vi "Scan action.vi"(0 "Index":i32, 1 "Channels: AO":T1={"AO amp (V)"=[0.002, 0.002, 0.002, 0.002, 0.002, 0.002, 0.002, 0.002], "AO DC (V)"=[0.0, 0.0, 0.0, 0.0, 0.0, 0.0, 0.0, 0.0], "AO f (Hz)"=[15.1, 15.11, 15.12, 15.13, 15.14, 15.15, 15.16, 15.17], "AO phi (deg)"=[0.0, 10.0, 20.0, 30.0, 40.0, 50.0, 60.0, 70.0], "function"=[enum."Sine Wave", enum."Sine Wave", enum."Sine Wave", enum."Sine Wave", enum."Sine Wave", enum."Sine Wave", enum."Sine Wave", enum."Sine Wave"]} {"AO f (Hz)" min=0.001 max=10000.0; "AO DC (V)" format="%#_6p"; "AO amp (V)" format="%#_6p"}, 2 "Scan control":T9=enum."DSA_Vamp", 3 "Scan Parameters":T8={"DAQ Channel"=2, "Label"="\nscaledVsg1=", "Start"=0.14, "End"=-0.060000000000000005, "Step"=-0.060000000000000005, "Rate"=-0.060000000000000005, "VISA resource name"=""} {"Rate" format="%.2f"; "Step" format="%#_6p"; "End" format="%#_6p"; "Start" format="%#_6p"}, 4 "Comments":string) -> (5 "Comments out":string, 6 "Channels: AO":T1={"AO amp (V)"=[0.002, 0.002, 0.002, 0.002, 0.002, 0.002, 0.002, 0.002], "AO DC (V)"=[0.0, 0.0, 0.0, 0.0, 0.0, 0.0, 0.0, 0.0], "AO f (Hz)"=[15.1, 15.11, 15.12, 15.13, 15.14, 15.15, 15.16, 15.17], "AO phi (deg)"=[0.0, 10.0, 20.0, 30.0, 40.0, 50.0, 60.0, 70.0], "function"=[enum."Sine Wave", enum."Sine Wave", enum."Sine Wave", enum."Sine Wave", enum."Sine Wave", enum."Sine Wave", enum."Sine Wave", enum."Sine Wave"]} {"AO f (Hz)" min=0.001 max=10000.0; "AO DC (V)" format="%#_6p"; "AO amp (V)" format="%#_6p"}, 7 "Stop?":bool)   [LabVIEW 2016, in "Transport.lvclass"]
uses:
  Transport.lvclass
  Typedefs/Enum - Action.ctl
  Typedefs/Cluster - ScanParamters.ctl
  <userlib>/LevyLab/Lockin-Multichannel/Typedefs/AO-cluster.ctl
  <userlib>/LevyLab/Lockin-Multichannel/Typedefs/AO_Amp-array.ctl
  <userlib>/LevyLab/Lockin-Multichannel/Typedefs/AO_DC-array.ctl
  <userlib>/LevyLab/Lockin-Multichannel/Typedefs/AO_f-array.ctl
  <userlib>/LevyLab/Lockin-Multichannel/Typedefs/AO_phi-array.ctl
  <userlib>/LevyLab/Lockin-Multichannel/Typedefs/Function-array.ctl
  <userlib>/LevyLab/Lockin-Multichannel/Typedefs/Function-enum.ctl
  <userlib>/LevyLab/Oxford 1820 API/Typedefs/Targets.ctl
  <userlib>/LevyLab/Oxford 1820 API/Mercury-1820-API.lvlib
panel:
  # "0"
  # "1"
  # "2"
  # "3"
  # "4"
  # "5"
  # "6"
  # "7"
  # "0"
  # "1"
  # "2"
  # "3"
  # "4"
  # "5"
  # "6"
  # "7"
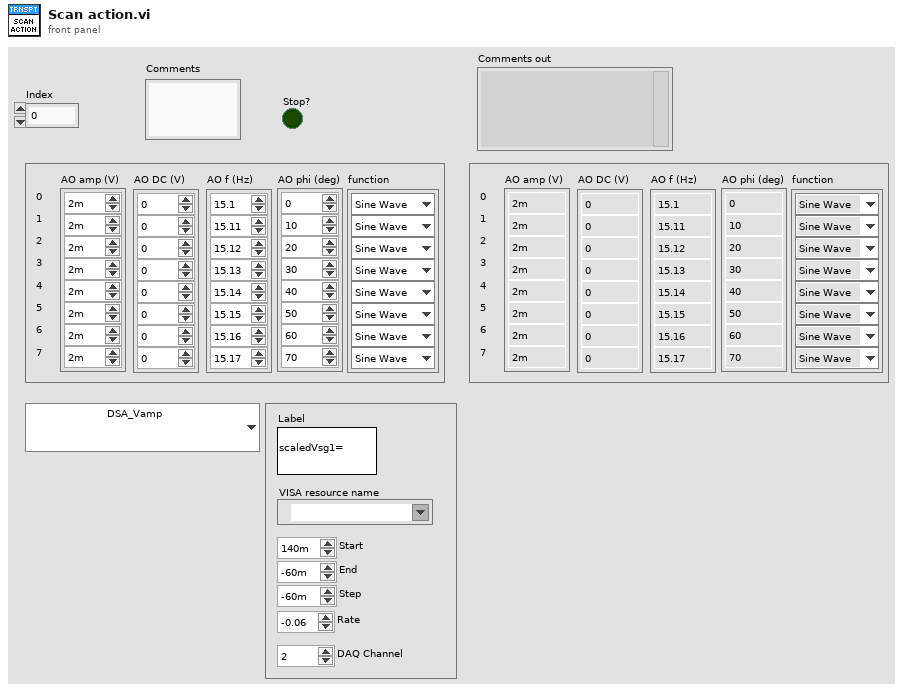
[diagram p1: front panel]
types:
  T1 = typedef "AO-cluster.ctl" = cluster{"AO amp (V)":T2, "AO DC (V)":T3, "AO f (Hz)":T4, "AO phi (deg)":T5, "function":T6}
  T2 = typedef "AO_Amp-array.ctl" = dbl[]
  T3 = typedef "AO_DC-array.ctl" = dbl[]
  T4 = typedef "AO_f-array.ctl" = dbl[]
  T5 = typedef "AO_phi-array.ctl" = dbl[]
  T6 = typedef "Function-array.ctl" = T7[]
  T7 = typedef "Function-enum.ctl" = enum16{"Sine Wave", "Triangle Wave", "Square Wave", "Sawtooth Wave"}
  T8 = typedef "Transport.lvclass/Cluster - ScanParamters.ctl" = cluster{"DAQ Channel":i32, "Label":string, "Start":dbl, "End":dbl, "Step":dbl, "Rate":dbl, "VISA resource name":refnum<visa-resource-name>}
  T9 = typedef "Transport.lvclass/Enum - Action.ctl" = enum16{"OFF", "DSA_Vamp", "DSA_freq", "DSA_Vsg1", "DSA_Vsg2", "DSA_Vsg3", "DAQ_Vbg", "B_Field", "Temp", "MW_freq1", "MW_freq2", "MW_amplitude1", "MW_amplitude2"}
  T10 = typedef "Mercury-1820-API.lvlib/Targets.ctl" = cluster{"Target Field (T)":dbl, "Target Field Rate (T/min)":dbl}
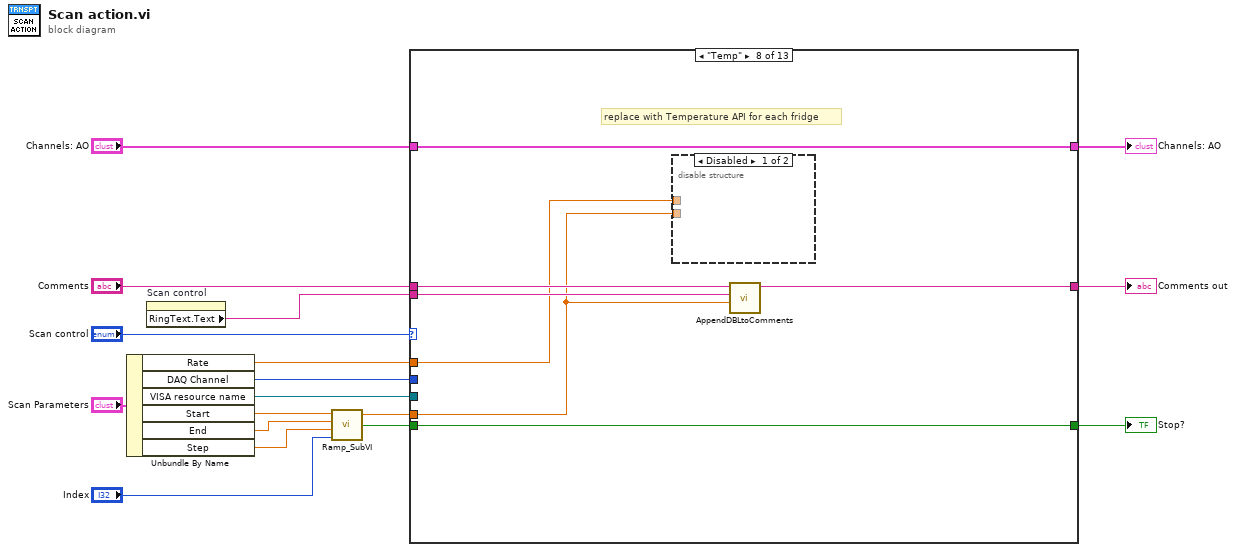
[diagram p0: block diagram]
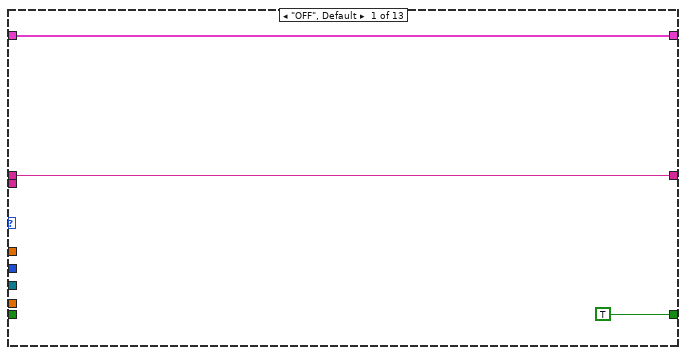
[diagram p2: hidden frame]
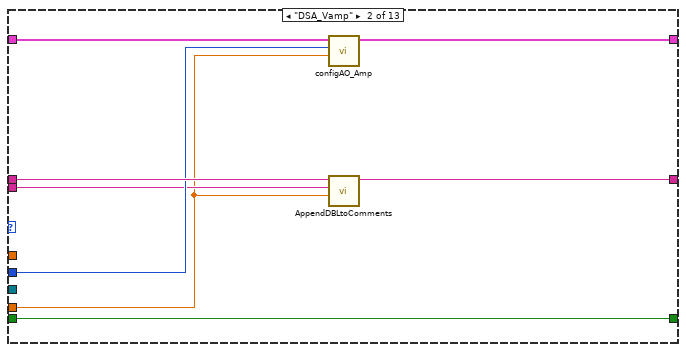
[diagram p3: hidden frame]
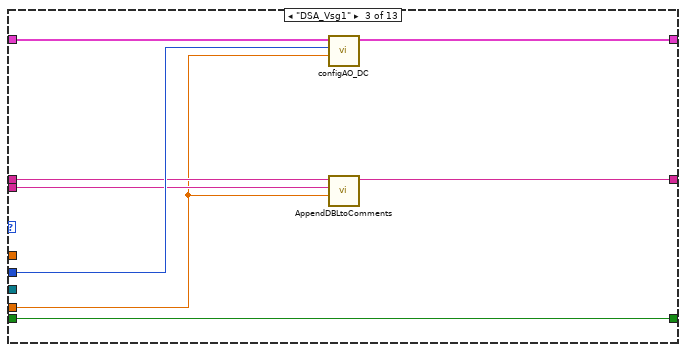
[diagram p4: hidden frame]
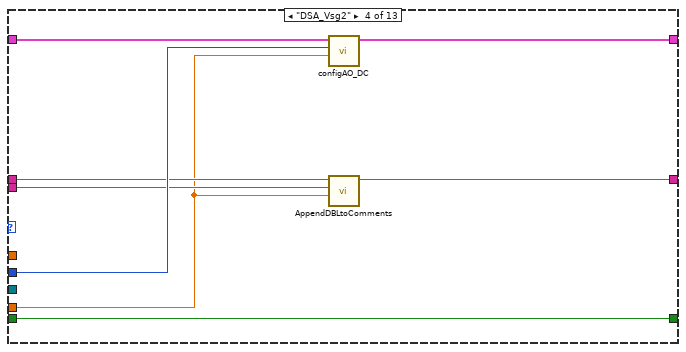
[diagram p5: hidden frame]
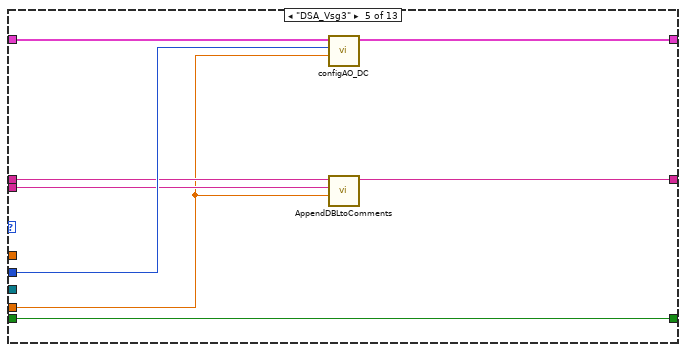
[diagram p6: hidden frame]
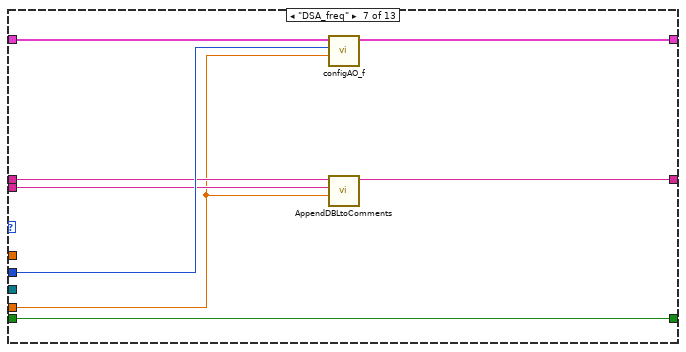
[diagram p8: hidden frame]
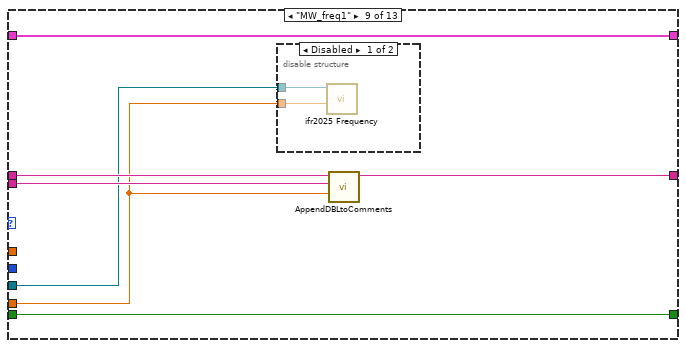
[diagram p10: hidden frame]
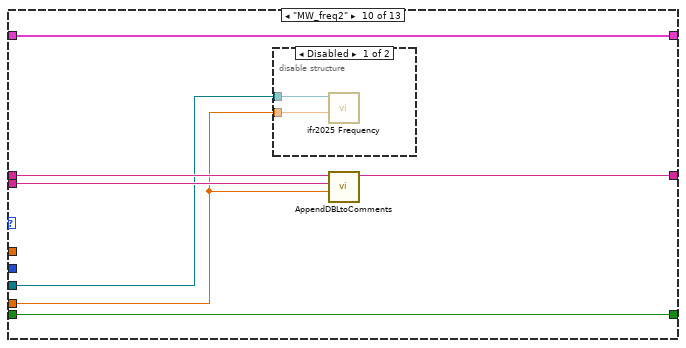
[diagram p12: hidden frame]
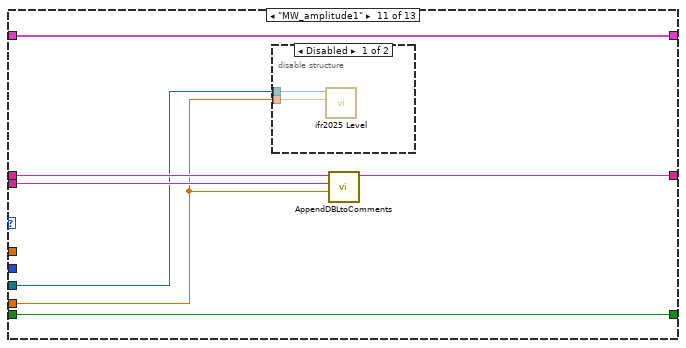
[diagram p14: hidden frame]
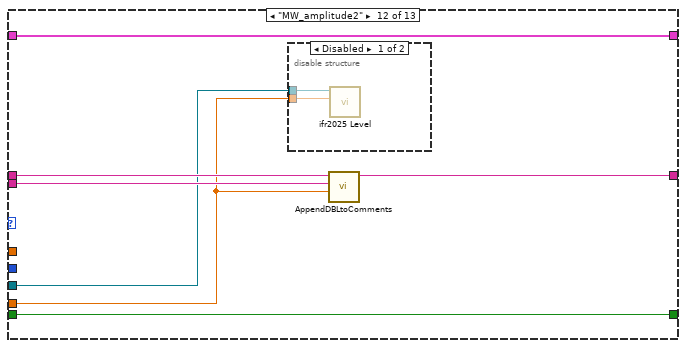
[diagram p16: hidden frame]
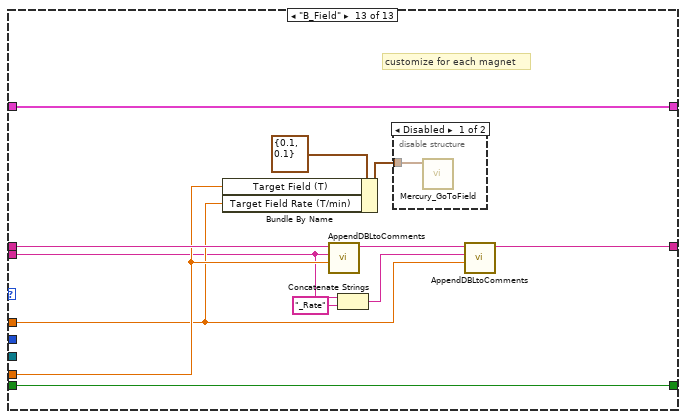
[diagram p18: hidden frame]
diagram:
  n1 = Unbundle By Name("Scan Parameters") -> ("Rate"=w9:dbl, "DAQ Channel"=w13:i32, "VISA resource name"=w1:refnum<visa-resource-name>, "Start"=w7:dbl, "End"=w6:dbl, "Step"=w5:dbl)
  n2 = property on="Scan control" class="Enum (strict)"() -> ("RingText.Text"=w8:string)  [unwired: 2 in, 2 out]
  n3 = call <userlib>:"Ramp_SubVI.vi"("index"="Index", "step"=w5, "end"=w6, "start"=w7) -> ("Stop?"=w3:bool, "Numeric"=w4:dbl)  [unwired: 1 in]
  n4 = case shown="\"Temp\"" "Scan control" {
    tunnel: w13 -> [_ w24 w34 w44 w52 _ w61 _ _ _ _ _ _]
    tunnel: "Comments" -> [w20 w28 w33 w41 w49 w54 w60 w69 w76 w85 w94 w103 w116]
    tunnel: w8 -> [_ w23 w31 w39 w47 _ w58 w67 w74 w83 w92 w101 w108]
    tunnel: [TRUE ("Stop?") w21 w29 w37 w45 w53 w56 w66 w73 w82 w91 w100 w115] -> w11
    tunnel: [w20 w27 w32 w40 w48 w54 w59 w68 w75 w84 w93 w102 w111] -> w10
    tunnel: "Channels: AO" -> [w18 w26 w36 w43 w51 w55 w63 w70 w77 w86 w95 w104 w113]
    tunnel: [w18 w25 w35 w42 w50 w55 w62 w70 w77 w86 w95 w104 w113] -> w15
    tunnel: w9 -> [_ _ _ _ _ _ _ w65 _ _ _ _ w110]
    tunnel: w4 -> [_ w22 w30 w38 w46 _ w57 w64 w72 w81 w90 w99 w114]
    tunnel: w3 -> [_ w21 w29 w37 w45 w53 w56 w66 w73 w82 w91 w100 w115]
    tunnel: w1 -> [_ _ _ _ _ _ _ _ w71 w80 w89 w98 _]
    frame "OFF", Default {
    }
    frame "DSA_Vamp" {
      n5 = call <userlib>:"configAO_Amp.vi"("new Amp (V)"=w22, "AO Channel"=w24, "Channels: AO"=w26) -> ("Channels: AO"=w25:T1)  [unwired: 7 in, 1 out]
      n6 = call "AppendDBLtoComments.vi"("Numeric"=w22, "Label"=w23, "Comments in"=w28) -> ("Comments out"=w27:string)  [unwired: 8 in]
    }
    frame "DSA_Vsg1" {
      n7 = call <userlib>:"configAO_DC.vi"("new DC (V)"=w30, "AO Channel"=w34, "Channels: AO"=w36) -> ("Channels: AO"=w35:T1)  [unwired: 7 in, 1 out]
      n8 = call "AppendDBLtoComments.vi"("Numeric"=w30, "Label"=w31, "Comments in"=w33) -> ("Comments out"=w32:string)  [unwired: 8 in]
    }
    frame "DSA_Vsg2" {
      n9 = call <userlib>:"configAO_DC.vi"("new DC (V)"=w38, "AO Channel"=w44, "Channels: AO"=w43) -> ("Channels: AO"=w42:T1)  [unwired: 7 in, 1 out]
      n10 = call "AppendDBLtoComments.vi"("Numeric"=w38, "Label"=w39, "Comments in"=w41) -> ("Comments out"=w40:string)  [unwired: 8 in]
    }
    frame "DSA_Vsg3" {
      n11 = call <userlib>:"configAO_DC.vi"("new DC (V)"=w46, "AO Channel"=w52, "Channels: AO"=w51) -> ("Channels: AO"=w50:T1)  [unwired: 7 in, 1 out]
      n12 = call "AppendDBLtoComments.vi"("Numeric"=w46, "Label"=w47, "Comments in"=w49) -> ("Comments out"=w48:string)  [unwired: 8 in]
    }
    frame "DAQ_Vbg" {
    }
    frame "DSA_freq" {
      n13 = call <userlib>:"configAO_f.vi"("new f (Hz)"=w57, "AO Channel"=w61, "Channels: AO"=w63) -> ("Channels: AO"=w62:T1)  [unwired: 7 in, 1 out]
      n14 = call "AppendDBLtoComments.vi"("Numeric"=w57, "Label"=w58, "Comments in"=w60) -> ("Comments out"=w59:string)  [unwired: 8 in]
    }
    frame "Temp" {
      # "replace with Temperature API for each fridge"
      n15 = disable-structure shown="Disabled" {
        disable-tunnel: w65 -> [_ _]
        disable-tunnel: w64 -> [_ _]
        frame Disabled {
        }
        frame Enabled {
        }
      }
      n16 = call "AppendDBLtoComments.vi"("Numeric"=w64, "Label"=w67, "Comments in"=w69) -> ("Comments out"=w68:string)  [unwired: 8 in]
    }
    frame "MW_freq1" {
      n17 = disable-structure shown="Disabled" {
        disable-tunnel: w72 -> [w79 _]
        disable-tunnel: w71 -> [w78 _]
        frame Disabled {
          n18 = call <instrlib>:"ifr2025 Frequency.vi"("Frequency (2.4E9)"=w79, "instrument handle"=w78) -> ()  [unwired: 8 in, 2 out]
        }
        frame Enabled {
        }
      }
      n19 = call "AppendDBLtoComments.vi"("Numeric"=w72, "Label"=w74, "Comments in"=w76) -> ("Comments out"=w75:string)  [unwired: 8 in]
    }
    frame "MW_freq2" {
      n20 = disable-structure shown="Disabled" {
        disable-tunnel: w81 -> [w88 _]
        disable-tunnel: w80 -> [w87 _]
        frame Disabled {
          n21 = call <instrlib>:"ifr2025 Frequency.vi"("Frequency (2.4E9)"=w88, "instrument handle"=w87) -> ()  [unwired: 8 in, 2 out]
        }
        frame Enabled {
        }
      }
      n22 = call "AppendDBLtoComments.vi"("Numeric"=w81, "Label"=w83, "Comments in"=w85) -> ("Comments out"=w84:string)  [unwired: 8 in]
    }
    frame "MW_amplitude1" {
      n23 = disable-structure shown="Disabled" {
        disable-tunnel: w90 -> [w97 _]
        disable-tunnel: w89 -> [w96 _]
        frame Disabled {
          n24 = call <instrlib>:"ifr2025 Level.vi"("RF Level (-137.0)"=w97, "instrument handle"=w96) -> ()  [unwired: 8 in, 2 out]
        }
        frame Enabled {
        }
      }
      n25 = call "AppendDBLtoComments.vi"("Numeric"=w90, "Label"=w92, "Comments in"=w94) -> ("Comments out"=w93:string)  [unwired: 8 in]
    }
    frame "MW_amplitude2" {
      n26 = disable-structure shown="Disabled" {
        disable-tunnel: w99 -> [w106 _]
        disable-tunnel: w98 -> [w105 _]
        frame Disabled {
          n27 = call <instrlib>:"ifr2025 Level.vi"("RF Level (-137.0)"=w106, "instrument handle"=w105) -> ()  [unwired: 8 in, 2 out]
        }
        frame Enabled {
        }
      }
      n28 = call "AppendDBLtoComments.vi"("Numeric"=w99, "Label"=w101, "Comments in"=w103) -> ("Comments out"=w102:string)  [unwired: 8 in]
    }
    frame "B_Field" {
      # "customize for each magnet"
      n29 = Bundle By Name(cluster=T10 {"Target Field (T)"=0.1, "Target Field Rate (T/min)"=0.1} ("Mercury Targets"), "Target Field (T)"=w114, "Target Field Rate (T/min)"=w110) -> (w117:T10)
      n30 = call "AppendDBLtoComments.vi"("Numeric"=w114, "Label"=w108, "Comments in"=w116) -> ("Comments out"=w112:string)  [unwired: 8 in]
      n31 = Concatenate Strings(w108, "_Rate" ("string")) -> (w107:string)
      n32 = disable-structure shown="Disabled" {
        disable-tunnel: w117 -> [w119 _]
        frame Disabled {
          n33 = call <userlib>:"Mercury_GoToField.vi"("Mercury Targets"=w119) -> ()  [unwired: 10 in, 1 out]
        }
        frame Enabled {
        }
      }
      n34 = call "AppendDBLtoComments.vi"("Numeric"=w110, "Label"=w107, "Comments in"=w112) -> ("Comments out"=w111:string)  [unwired: 8 in]
    }
  }
  "Comments out" <- w10
  "Stop?" <- w11
  "Channels: AO" <- w15
